vi "filename-generate-six-digit-thing.vi"() -> (1 "sixdigit":string, 2 "time":string, 3 "std date":string)   [LabVIEW 2018]
uses:
  <vilib>/regexp/Match Regular Expression.xnode
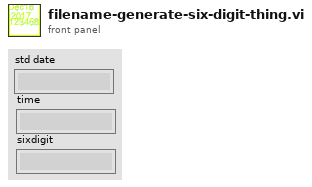
[diagram p1: front panel]
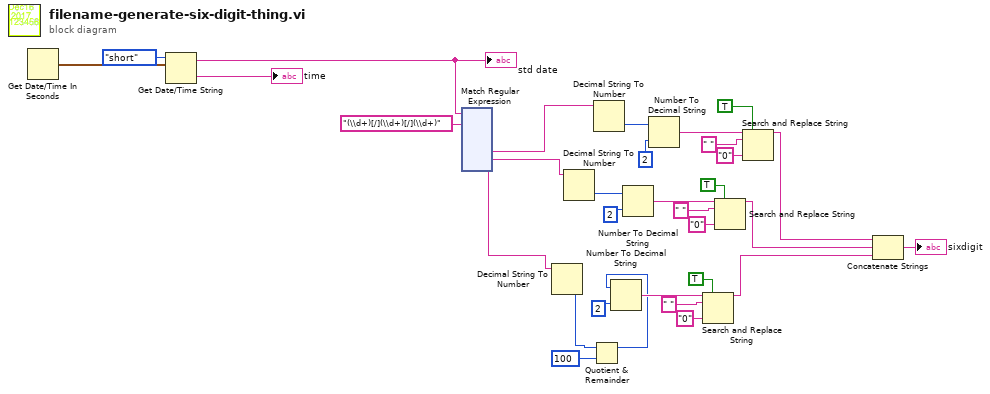
[diagram p0: block diagram]
diagram:
  n1 = Get Date/Time In Seconds() -> (seconds since 1Jan1904=w31:timestamp)
  n2 = Get Date/Time String(date format (0)=enum16{"short", "long", "abbreviated"}."short", seconds (now)=w31) -> (date string=w29:string, time string=→"time":string)  [unwired: 1 in]
  "std date" <- w29
  n3 = xnode "Match Regular Expression"("input string"=w29, "regular expression"="(\\d+)[/](\\d+)[/](\\d+)" ("regular expression (\"\")")) -> ("submatch 1"=w27:string, "submatch 2"=w16:string, "submatch 3"=w4:string)  [unwired: 4 in, 5 out]
  n4 = Decimal String To Number(string=w4) -> (number=w3:i32)  [unwired: 2 in, 1 out]
  n5 = Decimal String To Number(string=w16) -> (number=w10:i32)  [unwired: 2 in, 1 out]
  n6 = Quotient & Remainder(x=w3, y=100) -> (x-y*floor(x/y)=w2:i32)  [unwired: 1 out]
  n7 = Decimal String To Number(string=w27) -> (number=w14:i32)  [unwired: 2 in, 1 out]
  n8 = Number To Decimal String(number=w2, width (-)=i16 2) -> (decimal integer string=w6:string)
  n9 = Number To Decimal String(number=w10, width (-)=i16 2) -> (decimal integer string=w17:string)
  n10 = Number To Decimal String(number=w14, width (-)=i16 2) -> (decimal integer string=w22:string)
  n11 = Search and Replace String(replace all?=TRUE ("replace all? (F)"), input string=w6, search string=" ", replace string="0" ("replace string (\"\")")) -> (result string=w1:string)  [unwired: 4 in, 3 out]
  n12 = Search and Replace String(replace all?=TRUE ("replace all? (F)"), input string=w17, search string=" ", replace string="0" ("replace string (\"\")")) -> (result string=w15:string)  [unwired: 4 in, 3 out]
  n13 = Search and Replace String(replace all?=TRUE ("replace all? (F)"), input string=w22, search string=" ", replace string="0" ("replace string (\"\")")) -> (result string=w21:string)  [unwired: 4 in, 3 out]
  n14 = Concatenate Strings(w21, w15, w1) -> (→"sixdigit":string)
